vi "Initialization_CS4_ver1.0.vi"(0 "Magnet Control (CS4)":T1={"Action"=0, "Standby (s)"=0.0, "Heater on (s)"=300.0, "Sweep Setup "=[], "GPIB ADR"=0, "Change Para?"=FALSE} {"GPIB ADR" items=["None"=0, "10"=10]; "Sweep Setup"."Rate in Range (T/min)" min=0.001 max=0.5 step=0.001; "Sweep Setup"."Hold(min)" min=0.0; "Sweep Setup"."Set Point (T)" min=-9.0 max=9.0 step=0.001; "Action" items=["Up", "Down", "Pause", "Zero"]}, 2 "error in":errorcluster, 4 "First run?":bool) -> (1 "Set point":string, 3 "Hold(min)":dbl, 6 "B field Change?":bool, 7 "GPIB adr":string, 8 "Target B":string, 9 "Rate":string, 10 "error out":errorcluster)   [LabVIEW 2012]
panel:
  out "Display":string="+0.00000\r"
  out "Log":string
  # "Current\nField"
  # "T"
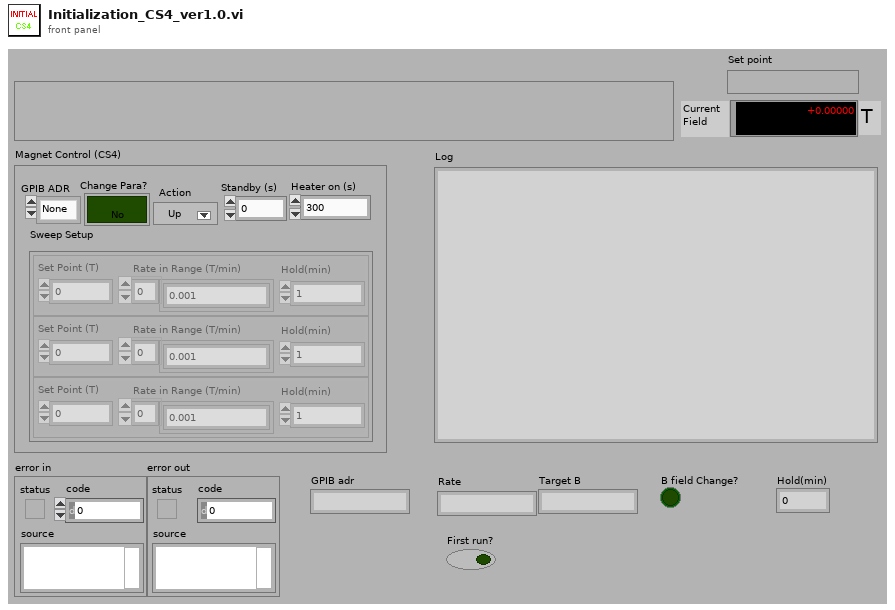
[diagram p1: front panel]
types:
  T1 = cluster{"Action":u16, "Standby (s)":dbl, "Heater on (s)":dbl, "Sweep Setup ":cluster{"Set Point (T)":dbl, "Hold(min)":dbl, "Rate in Range (T/min)":dbl[]}[], "GPIB ADR":u16, "Change Para?":bool}
  T2 = cluster{"Set Point (T)":dbl, "Hold(min)":dbl, "Rate in Range (T/min)":dbl[]}[]
  T3 = cluster{"Set Point (T)":dbl, "Hold(min)":dbl, "Rate in Range (T/min)":dbl[]}
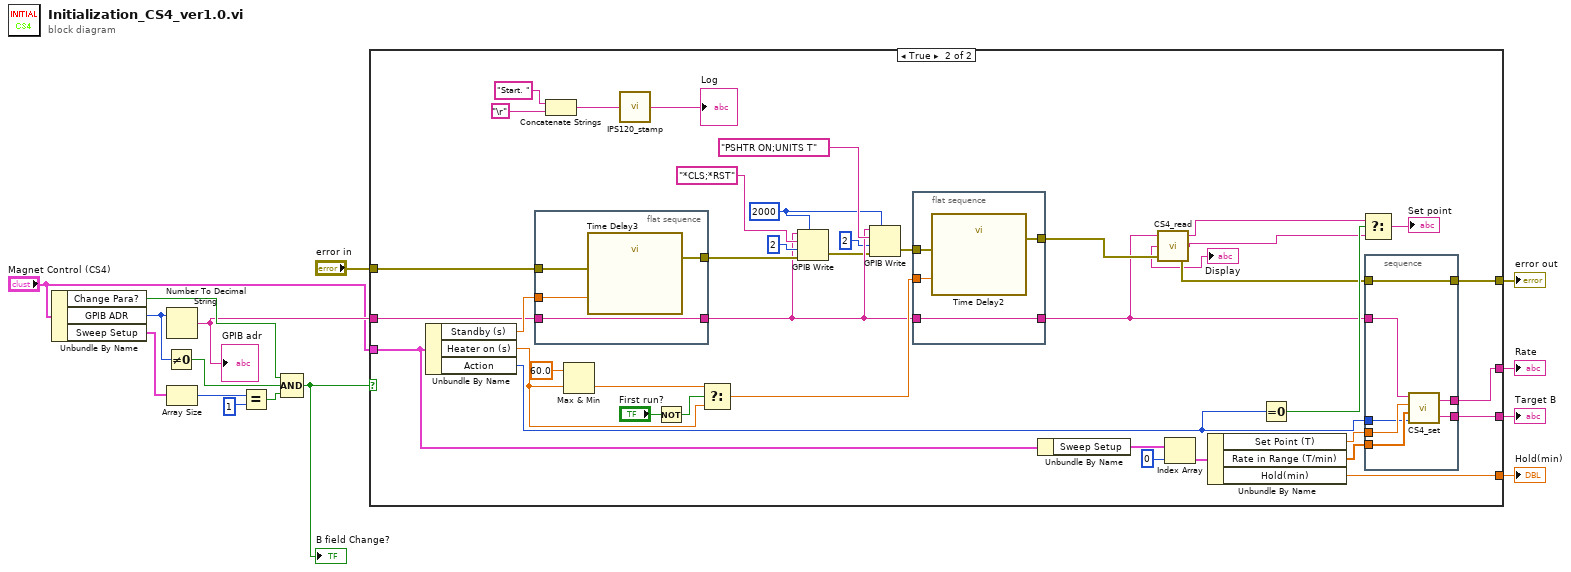
[diagram p0: block diagram]
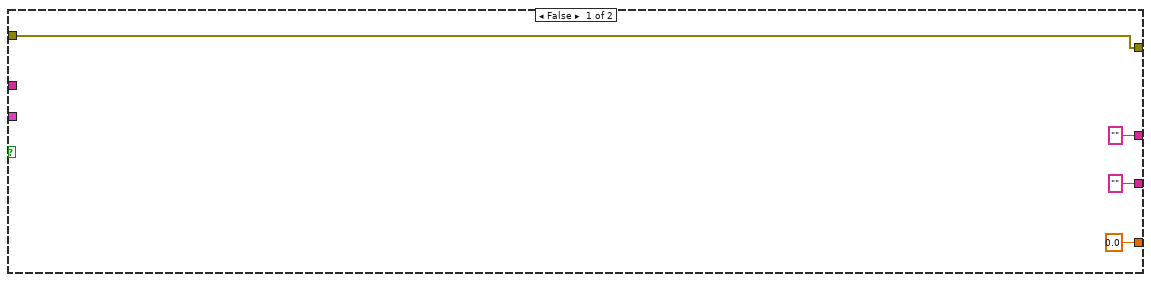
[diagram p2: hidden frame]
diagram:
  n1 = Unbundle By Name("Magnet Control (CS4)") -> ("Change Para?"=w9:bool, "GPIB ADR"=w3:u16, "Sweep Setup"=w13:T2)
  n2 = Not Equal To 0?(x=w3) -> (x != 0?=w8:bool)
  n3 = Number To Decimal String(number=w3) -> (decimal integer string=w2:string)  [unwired: 1 in]
  "GPIB adr" <- w2
  n4 = Array Size(array=w13) -> (size(s)=w12:i32)
  n5 = Equal?(x=w12, y=1) -> (x = y?=w7:bool)
  n6 = Compound Arithmetic op=AND(w9, w8, w7) -> (w10:bool)
  "B field Change?" <- w10
  n7 = case shown="True" w10 {
    tunnel: "Magnet Control (CS4)" -> [_ w50]
    tunnel: [w19 w27] -> w15
    tunnel: "error in" -> [w19 w53]
    tunnel: ["" ("Rate") w39] -> w6
    tunnel: ["" ("Target B") w38] -> w5
    tunnel: [0.0 ("Hold(min)") w49] -> w4
    tunnel: w2 -> [_ w42]
    frame False {
    }
    frame True {
      w29 = 2000 ("timeout ms (488.2 global)")
      n8 = Unbundle By Name(w50) -> ("Standby (s)"=w51:dbl, "Heater on (s)"=w45:dbl, "Action"=w36:u16)
      n9 = flat-sequence {
        tunnel: w51 -> [w71]
        tunnel: w53 -> [w70]
        tunnel: [w69] -> w33
        tunnel: w42 -> [w68]
        tunnel: [w68] -> w31
        frame #0 {
          n10 = call "Time Delay3"("error in (no error)"=w70, "Delay Time (s)"=w71) -> ("error out"=w69:errorcluster)  [unwired: 9 in]
        }
      }
      n11 = Concatenate Strings("Start. " ("Log"), "\r") -> (w58:string)
      n12 = Max & Min(x=60.0 ("t"), y=w45) -> (min(x,y)=w43:dbl)  [unwired: 1 out]
      n13 = call "IPS120_stamp.vi"("in"=w58) -> ("out"=→"Log":string)
      n14 = Not(x="First run?") -> (.not. x?=w44:bool)
      n15 = Select(t=w43, s=w44, f=w45) -> (s? t:f=w47:dbl)
      n16 = GPIB Write(0:w31, 1:"*CLS;*RST" ("data"), 2:i16 2 ("mode (0)"), 3:w33, 4:w29) -> (6:w26:errorcluster)  [unwired: 1 out]
      n17 = GPIB Write(0:w31, 1:"PSHTR ON;UNITS T" ("data"), 2:i16 2 ("mode (0)"), 3:w26, 4:w29) -> (6:w28:errorcluster)  [unwired: 1 out]
      n18 = flat-sequence {
        tunnel: w47 -> [w75]
        tunnel: w28 -> [w74]
        tunnel: [w73] -> w25
        tunnel: w31 -> [w72]
        tunnel: [w72] -> w22
        frame #0 {
          n19 = call "Time Delay2"("error in (no error)"=w74, "Delay Time (s)"=w75) -> ("error out"=w73:errorcluster)  [unwired: 9 in]
        }
      }
      n20 = Unbundle By Name(w50) -> ("Sweep Setup"=w56:T2)
      n21 = call "CS4_read.vi"("error in"=w25, "address string"=w22) -> ("error out"=w24:errorcluster, "Sweep Set point (Low)"=w20:string, "Sweep Set point (high)"=w21:string, "Real Field"=→"Display":string)
      n22 = Index Array(array=w56, index=0) -> (element=w54:T3)
      n23 = Unbundle By Name(w54) -> ("Set Point (T)"=w52:dbl, "Rate in Range (T/min)"=w40:dbl[], "Hold(min)"=w49:dbl)
      n24 = Equal To 0?(x=w36) -> (x = 0?=w37:bool)
      n25 = Select(t=w21, s=w37, f=w20) -> (s? t:f=→"Set point":string)
      n26 = stacked-sequence {
        tunnel: w52 -> [w67]
        tunnel: w40 -> [w66]
        tunnel: w22 -> [w65]
        tunnel: [w64] -> w39
        tunnel: [w63] -> w38
        tunnel: w36 -> [w62]
        tunnel: w24 -> [w61]
        tunnel: [w61] -> w27
        frame #0 {
          n27 = call "CS4_set.vi"("Action"=w62, "Rate in Range (T/min)"=w66, "Set Point"=w67, "GPIB add"=w65) -> ("Target B"=w63:string, "Rate"=w64:string)
        }
      }
    }
  }
  "error out" <- w15
  "Rate" <- w6
  "Target B" <- w5
  "Hold(min)" <- w4
